vi "TTA_Throw_User_Error.vi"(8 "error in":errorcluster, 9 "Error?":bool, 10 "Stop Execution on Fail":bool, 11 "Error Message":string) -> (0 "error out":errorcluster)   [LabVIEW 2016]
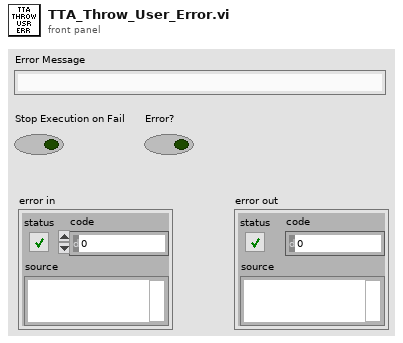
[diagram p1: front panel]
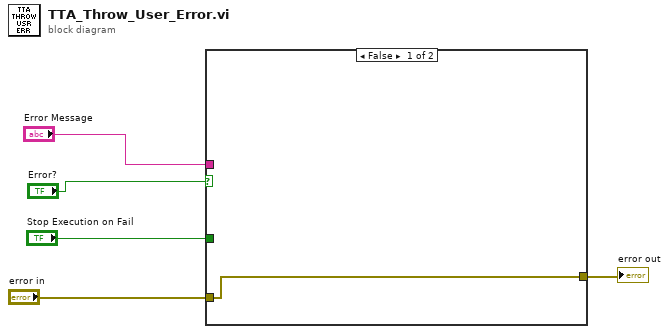
[diagram p0: block diagram]
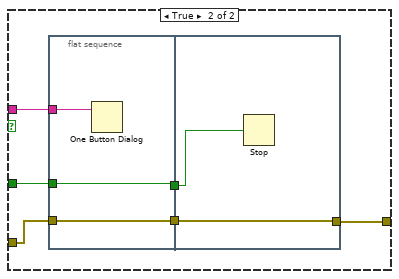
[diagram p2: hidden frame]
diagram:
  n1 = case shown="False" "Error?" {
    tunnel: "Stop Execution on Fail" -> [_ w11]
    tunnel: "Error Message" -> [_ w10]
    tunnel: "error in" -> [w6 w9]
    tunnel: [w6 w7] -> w1
    frame False {
    }
    frame True {
      n2 = flat-sequence {
        tunnel: w11 -> [w15]
        tunnel: [w15] -> w12
        tunnel: w10 -> [w14]
        tunnel: w9 -> [w13]
        tunnel: [w13] -> w8
        tunnel: w12 -> [w17]
        tunnel: w8 -> [w16]
        tunnel: [w16] -> w7
        frame #0 {
          n3 = One Button Dialog(message=w14) -> ()  [unwired: 1 in, 1 out]
        }
        frame #1 {
          n4 = Stop(stop? (T)=w17) -> ()
        }
      }
    }
  }
  "error out" <- w1
